vi "Test_3.vi"() -> ()   [LabVIEW 2015, in "Shore Library.lvlib"]
uses:
  Shore Library.lvlib
  Libraries/RDS Child Messages/MCB/MCB Motor Status.ctl
  Libraries/RDS Framework/RDS Message Class/RDS Message.lvclass
  Libraries/RDS Child Messages/MCB/MCB Status Message/MCB Status.lvclass
  Libraries/RDS Child Messages/MCB/MCB Status Message/MCB Status.lvclass/MCB Status.ctl
  Libraries/RDS Child Messages/RDS Child Messages.lvlib
panel:
  out "length 2":i32
  out "length":i32
  out "RDS Framework.lvlib:RDS Message.lvclass":refnum<class "RDS Message.lvclass">
  out "Motor Data":T1
  in  "output cluster":T1
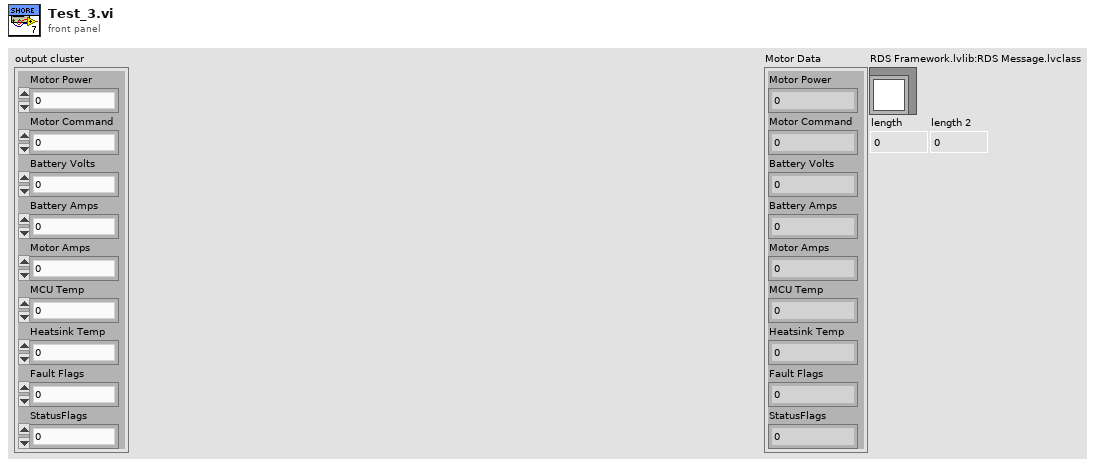
[diagram p1: front panel]
types:
  T1 = typedef "RDS Child Messages.lvlib/MCB Motor Status.ctl" = cluster{"Motor Power":i16, "Motor Command":i16, "Battery Volts":sgl, "Battery Amps":sgl, "Motor Amps":sgl, "MCU Temp":i16, "Heatsink Temp":i16, "Fault Flags":u16, "StatusFlags":u16}
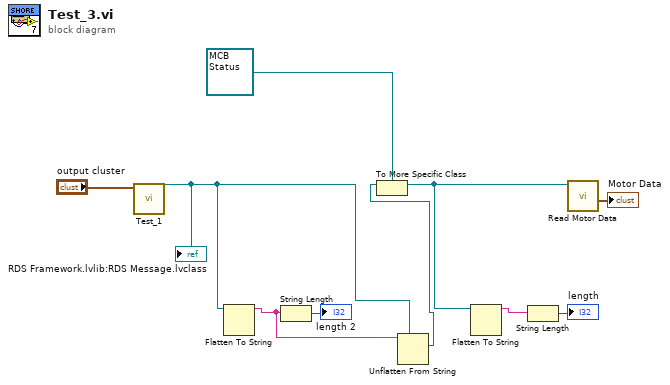
[diagram p0: block diagram]
diagram:
  n1 = call "Test_1.vi"("output cluster"="output cluster") -> ("RDS Framework.lvlib:RDS Message.lvclass"=w2:refnum<class "RDS Message.lvclass">)  [unwired: 10 in]
  "RDS Framework.lvlib:RDS Message.lvclass" <- w2
  n2 = Flatten To String(anything=w2) -> (data string=w3:string)  [unwired: 3 in, 2 out]
  n3 = String Length(string=w3) -> (length=→"length 2":i32)
  n4 = Unflatten From String(type=w2, binary string=w3) -> (value=w1:refnum<class "RDS Message.lvclass">)  [unwired: 3 in, 2 out]
  n5 = To More Specific Class(target class=refnum<class "MCB Status.lvclass"> refnum ("RDS Child Messages.lvlib:MCB Status.lvclass"), reference=w1) -> (specific class reference=w6:refnum<class "MCB Status.lvclass">)  [unwired: 1 in, 1 out]
  n6 = Flatten To String(anything=w6) -> (data string=w7:string)  [unwired: 3 in, 2 out]
  n7 = String Length(string=w7) -> (length=→"length":i32)
  n8 = call "Read Motor Data.vi"("MCB Status in"=w6) -> ("Motor Data"=→"Motor Data":T1)  [unwired: 7 in, 3 out]
